vi "BASE_Alarms.vi"(8 "error in (no error)":errorcluster, 9 "FAULT NUMBER":i32, 10 "STATUS":string, 11 "Ctl Refnum":refnum<vi>) -> (0 "error out":errorcluster)   [LabVIEW 2017]
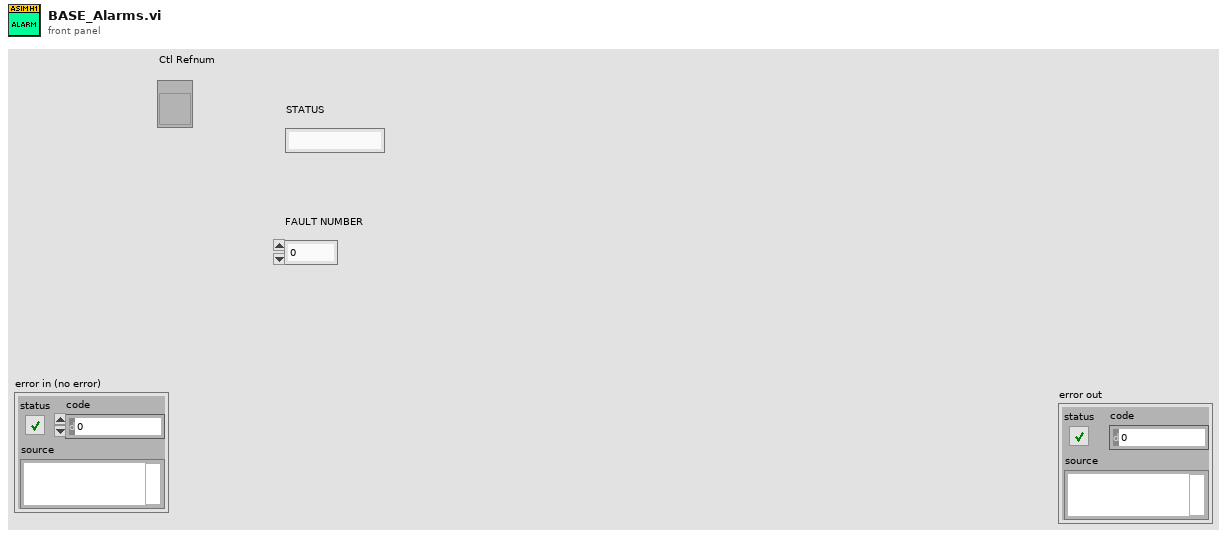
[diagram p1: front panel]
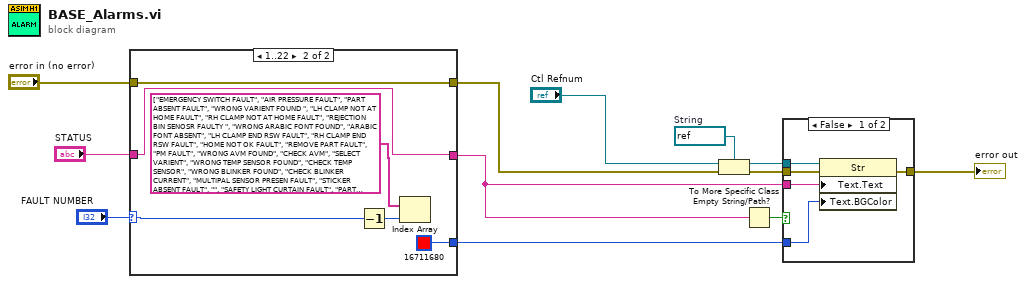
[diagram p0: block diagram]
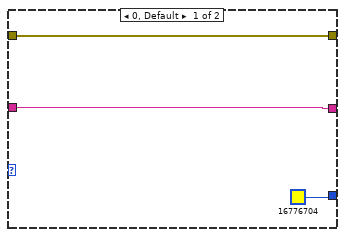
[diagram p3: hidden frame]
diagram:
  w12 = refnum<vi> refnum  # String
  n1 = case shown="1..22" "FAULT NUMBER" {
    selector: "FAULT NUMBER" -> [_ w20]
    tunnel: [w13 w16] -> w4
    tunnel: [u32 16776704 ("Color Box 2") u32 16711680 ("Color Box 2")] -> w6
    tunnel: [w14 w18] -> w3
    tunnel: "error in (no error)" -> [w14 w18]
    tunnel: "STATUS" -> [w13 w16]
    frame 0, Default {
    }
    frame 1..22 {
      n2 = Decrement(x=w20) -> (x-1=w21:i32)
      n3 = Index Array(array=string[] ["EMERGENCY SWITCH FAULT", "AIR PRESSURE FAULT", "PART ABSENT FAULT", "WRONG VARIENT FOUND ", "LH CLAMP NOT AT HOME FAULT", "RH CLAMP NOT AT HOME FAULT", "REJECTION BIN SENOSR FAULTY ", "WRONG ARABIC FONT FOUND", "ARABIC FONT ABSENT", "LH CLAMP END RSW FAULT", "RH CLAMP END RSW FAULT", "HOME NOT OK FAULT", "REMOVE PART FAULT", "PM FAULT", "WRONG AVM FOUND", "CHECK AVM", "SELECT VARIENT", "WRONG TEMP SENSOR FOUND", "CHECK TEMP SENSOR", "WRONG BLINKER FOUND", "CHECK BLINKER CURRENT", "MULTIPAL SENSOR PRESEN FAULT", "STICKER ABSENT FAULT", "", "SAFETY LIGHT CURTAIN FAULT", "PART REJECT FOR POWER FAILURE\nWRONG TOOL LIFE", "WRONG TOOL LIFE", "WRONG PART SCAN", "SCAN NOT DONE"], index=w21) -> ()  [unwired: 1 out]
    }
  }
  n4 = To More Specific Class(target class=w12, reference="Ctl Refnum", error in=w3) -> (specific class reference=w10:refnum<vi>, error out=w9:errorcluster)
  n5 = Empty String/Path?(string/path=w4) -> (empty?=w5:bool)
  n6 = case shown="False" w5 {
    tunnel: w10 -> [w26 _]
    tunnel: w9 -> [w25 w27]
    tunnel: [w24 w27] -> w8
    tunnel: w4 -> [w23 _]
    tunnel: w6 -> [w22 _]
    frame False {
      n7 = property class="Str"(reference=w26, error in=w25, "Text.Text"=w23, "Text.BGColor"=w22) -> (error out=w24:errorcluster)  [unwired: 1 out]
    }
    frame True {
    }
  }
  "error out" <- w8
